vi "Screen_to_3D.vi"(1 "X":dbl, 4 "Y":dbl) -> (8 "X_resolution":i16, 10 "Y_resolution":i16, 11 "Y_scaling":dbl, 14 "X_3D":dbl, 16 "Y_3D":dbl, 17 "Xmax":dbl=2.5, 19 "Ymax":dbl)   [LabVIEW 2011]
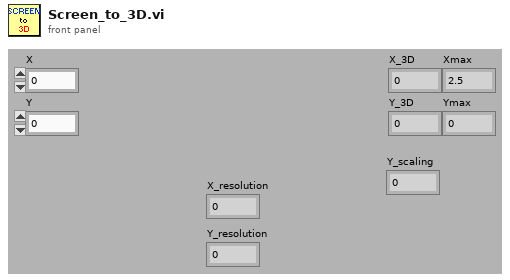
[diagram p1: front panel]
types:
  T1 = typedef "LVAllMonitorsDisplayTypeDef.ctl" = cluster{"Bounds":cluster{"Left":i16, "Top":i16, "Right":i16, "Bottom":i16}, "Depth":i16}[]
  T2 = cluster{"Bounds":cluster{"Left":i16, "Top":i16, "Right":i16, "Bottom":i16}, "Depth":i16}
  T3 = cluster{"Left":i16, "Top":i16, "Right":i16, "Bottom":i16}
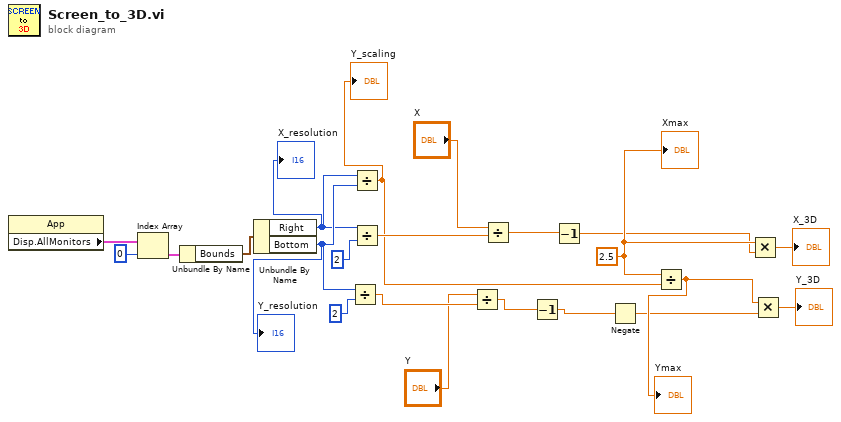
[diagram p0: block diagram]
diagram:
  w9 = 2.5 ("x")
  n1 = property class="App"() -> ("Disp.AllMonitors"=w20:T1)  [unwired: 2 in, 2 out]
  n2 = Index Array(array=w20, index=u16 0 ("Front Panel Window:Monitor")) -> (element=w22:T2)
  n3 = Unbundle By Name(w22) -> ("Bounds"=w19:T3)
  n4 = Unbundle By Name(w19) -> ("Right"=w17:i16, "Bottom"=w18:i16)
  "Y_resolution" <- w18
  "X_resolution" <- w17
  n5 = Divide(x=w18, y=i16 2) -> (x/y=w13:dbl)
  n6 = Divide(x=w17, y=w18) -> (x/y=w10:dbl)
  "Y_scaling" <- w10
  n7 = Divide(x=w17, y=i16 2) -> (x/y=w14:dbl)
  n8 = Divide(x="Y", y=w13) -> (x/y=w5:dbl)
  n9 = Divide(x="X", y=w14) -> (x/y=w2:dbl)
  n10 = Decrement(x=w5) -> (x-1=w4:dbl)
  n11 = Decrement(x=w2) -> (x-1=w1:dbl)
  n12 = Negate(x=w4) -> (-x=w7:dbl)
  n13 = Divide(x=w9, y=w10) -> (x/y=w8:dbl)
  "Ymax" <- w8
  n14 = Multiply(x=w9, y=w1) -> (x*y=→"X_3D":dbl)
  n15 = Multiply(x=w8, y=w7) -> (x*y=→"Y_3D":dbl)
  "Xmax" <- w9
